vi "saveAIA.vi"(0 "No Atoms":T1 format="%#_1f", 1 "Dark":T1, 2 "Atoms":T1, 3 "Db IN":string) -> (7 "error out":errorcluster)   [LabVIEW 2012]
uses:
  <vilib>/Analysis/Matrix/Datatypes/RealMatrix.ctl
  <vilib>/Analysis/Matrix/NI_Matrix.lvlib
panel:
  out "Entries in DB String":i32
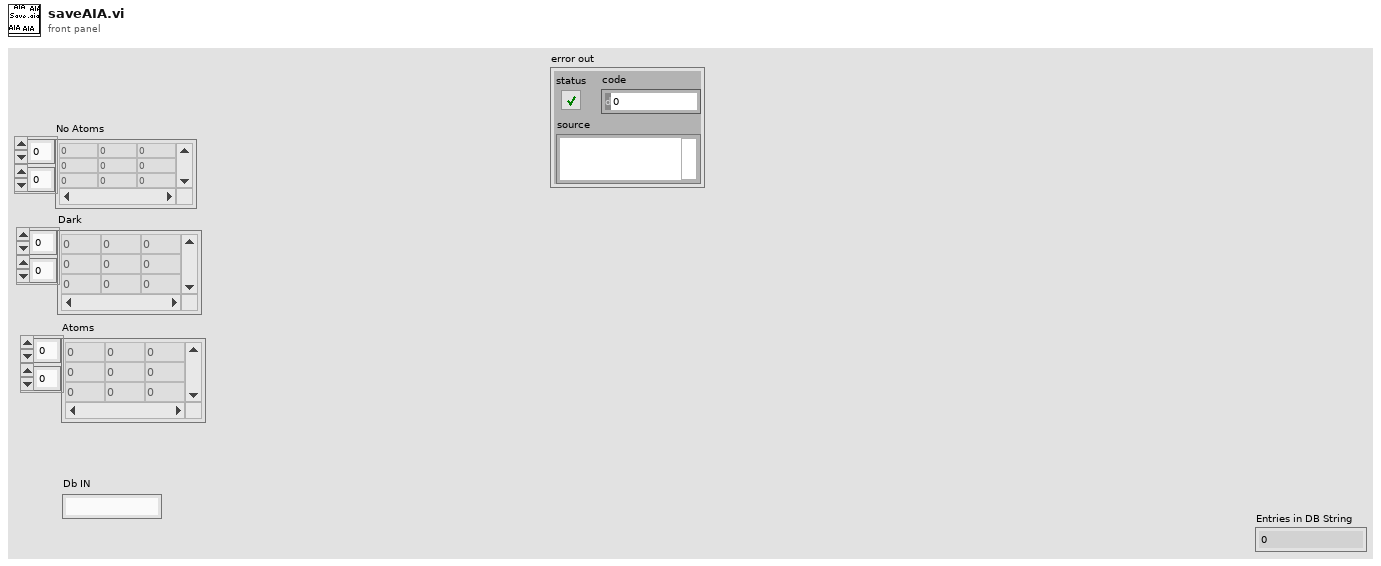
[diagram p1: front panel]
types:
  T1 = typedef "NI_Matrix.lvlib/RealMatrix.ctl" = dbl[][]
  T2 = enum16{"big-endian, network order", "native, host order", "little-endian"}
  T3 = enum16{"open", "replace", "create", "open or create", "replace or create", "replace or create with confirmation"}
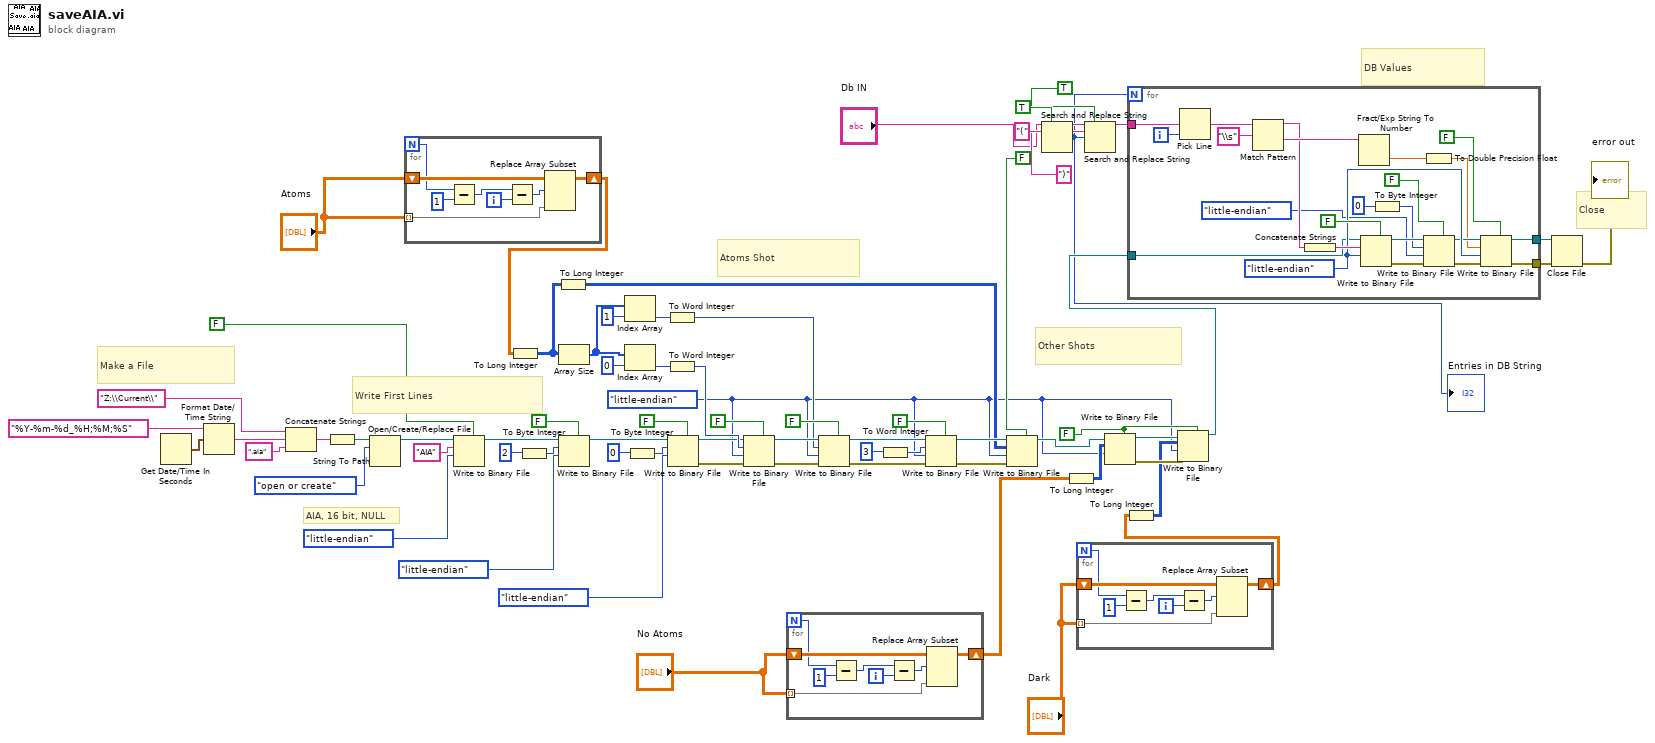
[diagram p0: block diagram]
diagram:
  w23 = FALSE ("prepend array or string size? (T)")
  w7 = T2."little-endian" ("byte order (0:big-endian, network order)")
  # "Close"
  # "DB Values"
  # "Other Shots"
  # "Atoms Shot"
  # "Write First Lines"
  # "Make a File"
  # "AIA, 16 bit, NULL"
  n1 = Get Date/Time In Seconds() -> (seconds since 1Jan1904=w70:timestamp)
  n2 = Format Date/Time String(time format string (%c)="%Y-%m-%d_%H;%M;%S", seconds (now)=w70) -> (date/time string=w69:string)  [unwired: 1 in]
  n3 = Concatenate Strings("Z:\\Current\\" ("string"), w69, ".aia" ("string")) -> (w65:string)
  n4 = String To Path(string=w65) -> (path=w64:path)
  n5 = Open/Create/Replace File(file path (use dialog)=w64, operation (0:open)=T3."open or create") -> (refnum out=w50:refnum<file>)  [unwired: 4 in, 2 out]
  n6 = for {
    N -> [w75]
    shift-right: [w76] -> w6
    shift-left: "Atoms" -> [w78]
    tunnel: "Atoms" -> [w77] mode=indexing
    i -> [w71]
    n7 = Subtract(x=w75, y=1) -> (x-y=w73:i32)
    n8 = Subtract(x=w73, y=w71) -> (x-y=w72:i32)
    n9 = Replace Array Subset(array=w78, new element=w77, index (row)=w72) -> (w76:T1)  [unwired: 1 in]
  }
  n10 = Write to Binary File(file (use dialog)=w50, data="AIA", 5:FALSE ("prepend array or string size? (T)"), 9:T2."little-endian" ("byte order (0:big-endian, network order)")) -> (refnum out=w60:refnum<file>)  [unwired: 2 in, 2 out]
  n11 = To Long Integer(number=w6) -> (32bit integer=w31:i32[][])
  n12 = To Byte Integer(number=2) -> (8bit integer=w53:i8)
  n13 = To Long Integer(number=w31) -> (32bit integer=w32:i32[][])
  n14 = Array Size(array=w31) -> (size(s)=w33:i32[])
  n15 = Write to Binary File(file (use dialog)=w60, data=w53, 5:FALSE ("prepend array or string size? (T)"), 9:T2."little-endian" ("byte order (0:big-endian, network order)")) -> (refnum out=w59:refnum<file>)  [unwired: 2 in, 2 out]
  n16 = Index Array(array=w33, index=1) -> (element=w37:i32)
  n17 = Index Array(array=w33, index=0) -> (element=w38:i32)
  n18 = To Byte Integer(number=0) -> (8bit integer=w51:i8)
  n19 = To Word Integer(number=w37) -> (16bit integer=w36:i16)
  n20 = To Word Integer(number=w38) -> (16bit integer=w39:i16)
  n21 = Write to Binary File(file (use dialog)=w59, data=w51, 5:FALSE ("prepend array or string size? (T)"), 9:T2."little-endian" ("byte order (0:big-endian, network order)")) -> (refnum out=w30:refnum<file>, error out=w29:errorcluster)  [unwired: 2 in, 1 out]
  n22 = Write to Binary File(file (use dialog)=w30, data=w39, error in=w29, 5:FALSE ("prepend array or string size? (T)"), 9:w7) -> (refnum out=w45:refnum<file>, error out=w28:errorcluster)  [unwired: 1 in, 1 out]
  n23 = for {
    N -> [w83]
    shift-right: [w84] -> w3
    shift-left: "No Atoms" -> [w86]
    tunnel: "No Atoms" -> [w85] mode=indexing
    i -> [w79]
    n24 = Subtract(x=w83, y=1) -> (x-y=w81:i32)
    n25 = Subtract(x=w81, y=w79) -> (x-y=w80:i32)
    n26 = Replace Array Subset(array=w86, new element=w85, index (row)=w80) -> (w84:T1)  [unwired: 1 in]
  }
  n27 = Write to Binary File(file (use dialog)=w45, data=w36, error in=w28, 5:FALSE ("prepend array or string size? (T)"), 9:w7) -> (refnum out=w44:refnum<file>, error out=w27:errorcluster)  [unwired: 1 in, 1 out]
  n28 = To Word Integer(number=3 ("index")) -> (16bit integer=w35:i16)
  n29 = Write to Binary File(file (use dialog)=w44, data=w35, error in=w27, 5:FALSE ("prepend array or string size? (T)"), 9:w7) -> (refnum out=w43:refnum<file>, error out=w26:errorcluster)  [unwired: 1 in, 1 out]
  n30 = Write to Binary File(file (use dialog)=w43, data=w32, error in=w26, 5:FALSE ("prepend array or string size? (T)"), 9:w7) -> (refnum out=w25:refnum<file>)  [unwired: 1 in, 2 out]
  n31 = Search and Replace String(replace all?=TRUE ("replace all? (F)"), input string="Db IN", search string="(") -> (result string=w18:string)  [unwired: 5 in, 3 out]
  n32 = To Long Integer(number=w3) -> (32bit integer=w24:i32[][])
  n33 = for {
    N -> [w91]
    shift-right: [w92] -> w1
    shift-left: "Dark" -> [w94]
    tunnel: "Dark" -> [w93] mode=indexing
    i -> [w87]
    n34 = Subtract(x=w91, y=1) -> (x-y=w89:i32)
    n35 = Subtract(x=w89, y=w87) -> (x-y=w88:i32)
    n36 = Replace Array Subset(array=w94, new element=w93, index (row)=w88) -> (w92:T1)  [unwired: 1 in]
  }
  n37 = Search and Replace String(replace all?=TRUE ("replace all? (F)"), input string=w18, search string=")") -> (result string=w14:string, number of replacements=w11:i32)  [unwired: 5 in, 2 out]
  "Entries in DB String" <- w11
  n38 = Write to Binary File(file (use dialog)=w25, data=w24, 5:w23, 9:w7) -> (refnum out=w22:refnum<file>, error out=w21:errorcluster)  [unwired: 2 in, 1 out]
  n39 = To Long Integer(number=w1) -> (32bit integer=w20:i32[][])
  n40 = Write to Binary File(file (use dialog)=w22, data=w20, error in=w21, 5:w23, 9:w7) -> (refnum out=w13:refnum<file>)  [unwired: 1 in, 2 out]
  n41 = for {
    N: w11 -> [_]
    tunnel: w14 -> [w116]
    tunnel: w13 -> [w97]
    tunnel: [w96] -> w12
    tunnel: [w95] -> w9
    i -> [w117]
    w105 = T2."little-endian" ("byte order (0:big-endian, network order)")
    n42 = Pick Line(multi-line string=w116, line index=w117) -> (output string=w115:string)  [unwired: 1 in]
    n43 = Match Pattern(string=w115, regular expression="\\s") -> (before substring=w108:string, after substring=w113:string)  [unwired: 1 in, 2 out]
    n44 = Concatenate Strings(w108) -> (w107:string)
    n45 = Fract/Exp String To Number(string=w113) -> (number=w102:dbl)  [unwired: 3 in, 1 out]
    n46 = Write to Binary File(file (use dialog)=w97, data=w107, 5:FALSE ("prepend array or string size? (T)"), 9:w105) -> (refnum out=w109:refnum<file>, error out=w110:errorcluster)  [unwired: 2 in, 1 out]
    n47 = To Byte Integer(number=0) -> (8bit integer=w99:i8)
    n48 = To Double Precision Float(number=w102) -> (double precision float=w100:dbl)
    n49 = Write to Binary File(file (use dialog)=w109, data=w99, error in=w110, 5:FALSE ("prepend array or string size? (T)"), 9:T2."little-endian" ("byte order (0:big-endian, network order)")) -> (refnum out=w103:refnum<file>, error out=w106:errorcluster)  [unwired: 1 in, 1 out]
    n50 = Write to Binary File(file (use dialog)=w103, data=w100, error in=w106, 5:FALSE ("prepend array or string size? (T)"), 9:w105) -> (refnum out=w96:refnum<file>, error out=w95:errorcluster)  [unwired: 1 in, 1 out]
  }
  n51 = Close File(refnum=w12, error in=w9) -> (error out=→"error out":errorcluster)  [unwired: 1 out]
